vi "ni579x FPGA Align.vi"(0 "sync.resources":T1, 1 "sync.meas.Reference Clock":refnum<k21>, 2 "sync.meas.FPGA Clock x2":refnum<k21>) -> (4 "sync.resources":T1)   [LabVIEW 2013, in "ni579x Synchronization v1 FPGA.lvlib"]
doc: "*** THIS VI IS DEPRECATED. USE ni579x FPGA Align 2.vi ***\n\nAlign the targets participating in synchronization. This must occur before a signal can be synchronized.\n\nThere are two flavors of alignment to chose from -- Host Align and FPGA Align. The two flavors produce the same quality of synchronization, but differ in requirements and versatility of operation.\n\nWhen using <B>ni579x FPGA Align</B>, the Single Cycle Timed Loop (SCTL) rate (that this VI is in) must be an integer multiple of the <B>sync.cptr.Reference Clock</B> rate, and the SCTL clock must have a fixed phase relationship to the reference clock. Each target performs its alignment independently, so FPGA Align does not require an FPGA I/O line. It's also possible to use FPGA Align without host interaction. FPGA Align has 100% repeatability if-and-only-if the target-to-target phase relationship is low and does not change.\n\nWhen using <B>ni579x Host Align</B>, the SCTL rate may be arbitrary (yet still must have a fixed phase relationship to the other targets). The CPTR period may also be arbitrary. This alignment process is coordinated by the host, and requires an FPGA I/O line for orchestration. Host Align has 100% repeatability; if the hardware configuration remains constant, so will the level of synchronization.\n\n<B>Input Parameters</B>\n\n<B>sync.resources</B> identifies the Synchronization instance. 'sync.resources' is obtained from the ni579x Create VI of this library.\n\n<B>sync.meas.Reference Clock</B> is used by the measurement logic as the \"start\" signal.\n\nWhen using 'ni579x FPGA Align', the 'sync.meas.Reference Clock' must be the same clock that the target's FPGA Clock is locked to. This is commonly PXI_Clk10.\n\n<B>sync.meas.FPGA Clock x2</B> is used by the measurement logic as the measurement clock. This clock must run at twice the rate of the FPGA Clock (the clock that drives the Single Cycle Timed Loop (SCTL) which this VI is in). This clock must also be derrived from the FPGA Clock, so that it has a fixed phase relationship. This is commonly IO Module\\Sample Clock x2.\n\n<B>Output Parameters</B>\n\n<B>sync.resources</B> is the same instance that was passed in for 'sync.resources'."
uses:
  <instrlib>/ni579x/Synchronization/v1/FPGA/ni579x Synchronization v1 FPGA.lvlib
  <instrlib>/ni579x/Synchronization/v1/FPGA/Implementation/Resources.ctl
  <vilib>/rvi/eio/common/nirviEmuTemplateMethod_errors.vi
  <vilib>/eio/EIONode/EIONode.xnode
  <instrlib>/_niInstr/Basic Elements/v1/FPGA/niInstr Basic Elements v1 FPGA.lvlib
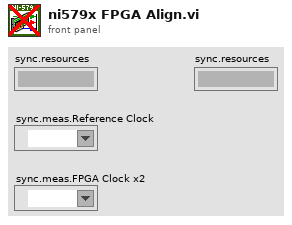
[diagram p1: front panel]
types:
  T1 = typedef "ni579x Synchronization v1 FPGA.lvlib/Resources.ctl" = cluster{"master":refnum<k21>, "meas.enable":refnum<k21>, "meas.ready":refnum<k21>, "meas.arm":refnum<k21>, "meas.valid":refnum<k21>, "meas.value":refnum<k21>, "meas.oversample clock":refnum<k21>, "meas.oversample factor":refnum<k21>, "cptr":refnum<k21>, "cptr.adjust":refnum<k21>, "cptr.period":refnum<k21>}
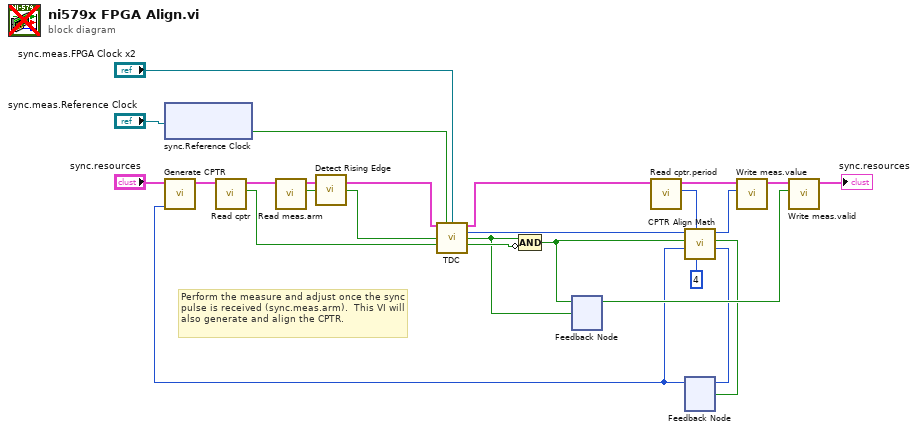
[diagram p0: block diagram]
diagram:
  # "Perform the measure and adjust once the sync pulse is received (sync.meas.arm).  This VI will also generate and align the CPTR."
  n1 = xnode ("sync.Reference Clock")("FPGA I/O In"="sync.meas.Reference Clock") -> ("I/O Item"=w20:bool)  [unwired: 1 out]
  n2 = feedback #1() -> (w25:bool)  [unwired: 1 in]
  n3 = feedback #2() -> (w15:u16)  [unwired: 1 in]
  n4 = call <instrlib>:"Generate CPTR.vi"("sync.cptr.adjust"=w15, "sync.resources"="sync.resources") -> ("sync.resources"=w16:T1)  [unwired: 9 in]
  n5 = call <instrlib>:"Read cptr.vi"("sync.resources"=w16) -> ("cptr"=w17:bool, "sync.resources"=w18:T1)  [unwired: 9 in]
  n6 = call <instrlib>:"Read meas.arm.vi"("sync.resources"=w18) -> ("meas.arm"=w23:bool, "sync.resources"=w5:T1)  [unwired: 9 in]
  n7 = call <instrlib>:"Detect Rising Edge.vi"("signal"=w23) -> ("edge detected"=w19:bool)  [unwired: 14 in]
  n8 = call <instrlib>:"TDC.vi"("sync.resources"=w5, "sync.Reference Clock"=w20, "sync.meas.oversample clock"="sync.meas.FPGA Clock x2", "sync.meas.arm"=w19, "sync.cptr"=w17) -> ("sync.resources"=w6:T1, "count out"=w11:u16, "count valid"=w21:bool, "rollover error"=w22:bool)  [unwired: 6 in, 1 out]
  n9 = Compound Arithmetic op=AND(w21, invert w22) -> (w10:bool)
  n10 = feedback-in #1(w10, w21) -> ()
  n11 = call <instrlib>:"Read cptr.period.vi"("sync.resources"=w6) -> ("cptr.period"=w8:u16, "sync.resources"=w9:T1)  [unwired: 9 in]
  n12 = call <instrlib>:"CPTR Align Math.vi"("sync.meas.oversample factor"=u16 4, "sync.cptr.period"=w8, "sync.cptr.adjust"=w15, "measurement valid"=w10, "measurement"=w11) -> ("new sync.cptr.adjust"=w14:u16, "new sync.cptr.adjust valid"=w4:bool, "measurement (in sample clocks)"=w12:u16)  [unwired: 4 in]
  n13 = feedback-in #2(w14, w4) -> ()
  n14 = call <instrlib>:"Write meas.value.vi"("meas.value"=w12, "sync.resources"=w9) -> ("sync.resources"=w13:T1)  [unwired: 9 in]
  n15 = call <instrlib>:"Write meas.valid.vi"("meas.valid"=w25, "sync.resources"=w13) -> ("sync.resources"=→"sync.resources":T1)  [unwired: 9 in]
